vi "convert spotfield to WF.vi"(8 "error in (no error)":errorcluster, 10 "TDK-Lambda Z in":refnum<class "ThorlabsWFS.lvclass">, 11 "VISA Refnum in":refnum<visa-resource-name>) -> (0 "error out":errorcluster, 1 "output cluster":T1, 2 "Array Wavefront":sgl[](array[numeric]), 3 "VISA Refnum out":refnum<visa-resource-name>)   [LabVIEW 2020, in "ThorlabsWFS.lvclass"]
uses:
  ThorlabsWFS.lvclass
  analysis result.ctl
  OnOffTypeDef.ctl
  ThorlabsWFS.lvclass/ThorlabsWFS.ctl
panel:
  in  "analysis result":T1
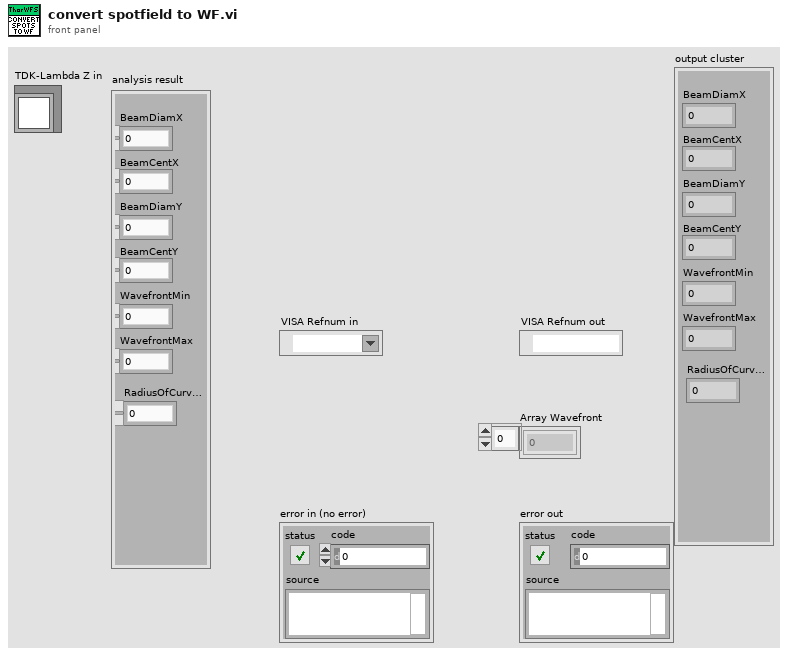
[diagram p1: front panel]
types:
  T1 = typedef "ThorlabsWFS.lvclass/analysis result.ctl" = cluster{"BeamDiamX":dbl, "BeamCentX":dbl, "BeamDiamY":dbl, "BeamCentY":dbl, "WavefrontMin":dbl, "WavefrontMax":dbl, "RadiusOfCurvature":dbl}
  T2 = typedef "OnOffTypeDef.ctl" = enum16{"off", "on"}
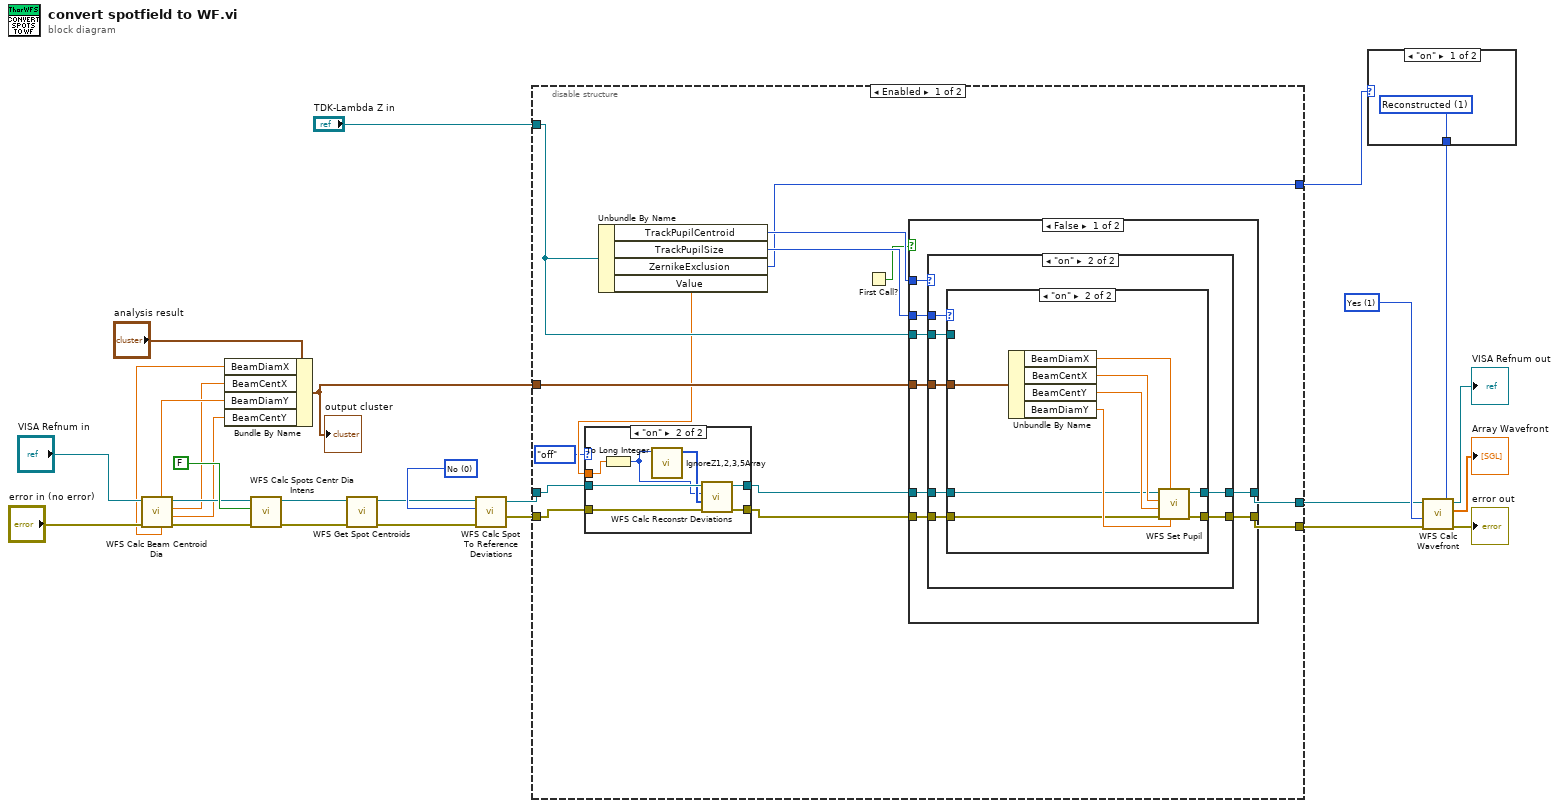
[diagram p0: block diagram]
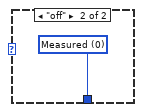
[diagram p2: hidden frame]
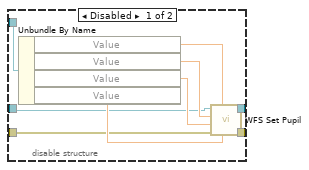
[diagram p5: hidden frame]
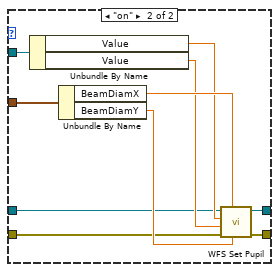
[diagram p6: hidden frame]
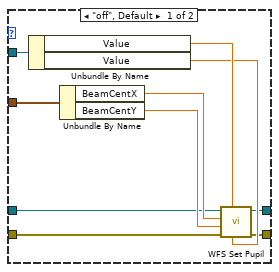
[diagram p7: hidden frame]
diagram:
  w25 = 1 items=["Yes"=1, "No"=0] ("Limit to Pupil (No)")
  w22 = 0 items=["No", "Yes"] ("Cancel Wavefront Tilt (No)")
  n1 = call "WFS Calc Beam Centroid Dia.vi"("error in (no error)"="error in (no error)", "instrument handle"="VISA Refnum in") -> ("error out"=w13:errorcluster, "Beam Centroid Y mm"=w9:dbl, "Beam Centroid X mm"=w8:dbl, "instrument handle out"=w12:refnum<visa-resource-name>, "Beam Diameter X mm"=w10:dbl, "Beam Diameter Y mm"=w11:dbl)  [unwired: 4 in]
  n2 = Bundle By Name(cluster="analysis result", "BeamDiamX"=w10, "BeamCentX"=w8, "BeamDiamY"=w11, "BeamCentY"=w9) -> (w7:T1)
  "output cluster" <- w7
  n3 = call "WFS Calc Spots Centr Dia Intens.vi"("error in (no error)"=w13, "Dynamic Noise Cut (On)"=FALSE, "instrument handle"=w12) -> ("error out"=w18:errorcluster, "instrument handle out"=w17:refnum<visa-resource-name>)  [unwired: 7 in]
  n4 = call "WFS Get Spot Centroids.vi"("error in (no error)"=w18, "instrument handle"=w17) -> ("error out"=w21:errorcluster, "instrument handle out"=w20:refnum<visa-resource-name>)  [unwired: 6 in, 2 out]
  n5 = call "WFS Calc Spot To Reference Deviations.vi"("error in (no error)"=w21, "Cancel Wavefront Tilt (No)"=w22, "instrument handle"=w20) -> ("error out"=w3:errorcluster, "instrument handle out"=w5:refnum<visa-resource-name>)  [unwired: 7 in]
  n6 = disable-structure shown="Enabled" {
    disable-tunnel: w7 -> [w38 _]
    disable-tunnel: "TDK-Lambda Z in" -> [w37 _]
    disable-tunnel: w5 -> [w34 w121]
    disable-tunnel: [w36 w121] -> w4
    disable-tunnel: w3 -> [w33 w120]
    disable-tunnel: [w35 w120] -> w2
    disable-tunnel: [w29 _] -> w1
    frame Enabled {
      n7 = Unbundle By Name(w37) -> ("TrackPupilCentroid"=w41:T2, "TrackPupilSize"=w40:T2, "ZernikeExclusion"=w29:T2, "Value"=w30:dbl)
      n8 = case shown="\"on\"" OnOffTypeDef."off" ("IgnoreZ1,2,3,5") {
        tunnel: w34 -> [w43 w50]
        tunnel: w33 -> [w42 w49]
        tunnel: [w42 w48] -> w32
        tunnel: [w43 w47] -> w31
        tunnel: w30 -> [_ w45]
        frame "off", Default {
        }
        frame "on" {
          n9 = To Long Integer(number=w45) -> (32bit integer=w44:i32)
          n10 = call "IgnoreZ1,2,3,5Array.vi"("Zernike Order"=w44) -> ("output array"=w46:i32[])  [unwired: 10 in]
          n11 = call "WFS Calc Reconstr Deviations.vi"("error in (no error)"=w49, "Array Zernike Reconstruct"=w46, "Zernike Orders"=w44, "instrument handle"=w50) -> ("error out"=w48:errorcluster, "instrument handle out"=w47:refnum<visa-resource-name>)  [unwired: 4 in, 2 out]
        }
      }
      n12 = First Call?() -> (First Call?: T/F=w39:bool)
      n13 = case shown="False" w39 {
        tunnel: w41 -> [w58 _]
        tunnel: w40 -> [w57 _]
        tunnel: w38 -> [w56 _]
        tunnel: w37 -> [w55 _]
        tunnel: w31 -> [w54 w119]
        tunnel: [w53 w119] -> w36
        tunnel: w32 -> [w52 w118]
        tunnel: [w51 w118] -> w35
        frame False {
          n14 = case shown="\"on\"" w58 {
            tunnel: w57 -> [w65 w98]
            tunnel: w56 -> [w64 w97]
            tunnel: w55 -> [w63 w96]
            tunnel: w54 -> [w62 w95]
            tunnel: [w61 w94] -> w53
            tunnel: w52 -> [w60 w93]
            tunnel: [w59 w92] -> w51
            frame "off", Default {
              n15 = case shown="\"off\", Default" w65 {
                tunnel: w64 -> [_ w91]
                tunnel: w63 -> [w70 w88]
                tunnel: w62 -> [w69 w85]
                tunnel: [w68 w84] -> w61
                tunnel: w60 -> [w67 w83]
                tunnel: [w66 w82] -> w59
                frame "off", Default {
                  n16 = disable-structure shown="Enabled" {
                    disable-tunnel: w70 -> [w79 _]
                    disable-tunnel: w69 -> [w74 w81]
                    disable-tunnel: [w73 w81] -> w68
                    disable-tunnel: w67 -> [w72 w80]
                    disable-tunnel: [w71 w80] -> w66
                    frame Disabled {
                      n17 = Unbundle By Name(w79) -> ("Value"=w78:dbl, "Value"=w76:dbl, "Value"=w75:dbl, "Value"=w77:dbl)
                      n18 = call "WFS Set Pupil.vi"("Pupil Diameter Y mm"=w77, "Pupil Diameter X mm"=w78, "error in (no error)"=w72, "Pupil Center Y mm"=w75, "Pupil Center X mm"=w76, "instrument handle"=w74) -> ("error out"=w71:errorcluster, "instrument handle out"=w73:refnum<visa-resource-name>)  [unwired: 4 in]
                    }
                    frame Enabled {
                    }
                  }
                }
                frame "on" {
                  n19 = Unbundle By Name(w88) -> ("Value"=w87:dbl, "Value"=w86:dbl)
                  n20 = Unbundle By Name(w91) -> ("BeamDiamX"=w90:dbl, "BeamDiamY"=w89:dbl)
                  n21 = call "WFS Set Pupil.vi"("Pupil Diameter Y mm"=w89, "Pupil Diameter X mm"=w90, "error in (no error)"=w83, "Pupil Center Y mm"=w86, "Pupil Center X mm"=w87, "instrument handle"=w85) -> ("error out"=w82:errorcluster, "instrument handle out"=w84:refnum<visa-resource-name>)  [unwired: 4 in]
                }
              }
            }
            frame "on" {
              n22 = case shown="\"on\"" w98 {
                tunnel: w97 -> [w106 w117]
                tunnel: w96 -> [w105 _]
                tunnel: w95 -> [w102 w109]
                tunnel: [w101 w112] -> w94
                tunnel: w93 -> [w100 w110]
                tunnel: [w99 w111] -> w92
                frame "off", Default {
                  n23 = Unbundle By Name(w105) -> ("Value"=w104:dbl, "Value"=w103:dbl)
                  n24 = Unbundle By Name(w106) -> ("BeamCentX"=w108:dbl, "BeamCentY"=w107:dbl)
                  n25 = call "WFS Set Pupil.vi"("Pupil Diameter Y mm"=w103, "Pupil Diameter X mm"=w104, "error in (no error)"=w100, "Pupil Center Y mm"=w107, "Pupil Center X mm"=w108, "instrument handle"=w102) -> ("error out"=w99:errorcluster, "instrument handle out"=w101:refnum<visa-resource-name>)  [unwired: 4 in]
                }
                frame "on" {
                  n26 = Unbundle By Name(w117) -> ("BeamDiamX"=w116:dbl, "BeamCentX"=w115:dbl, "BeamCentY"=w113:dbl, "BeamDiamY"=w114:dbl)
                  n27 = call "WFS Set Pupil.vi"("Pupil Diameter Y mm"=w114, "Pupil Diameter X mm"=w116, "error in (no error)"=w110, "Pupil Center Y mm"=w113, "Pupil Center X mm"=w115, "instrument handle"=w109) -> ("error out"=w111:errorcluster, "instrument handle out"=w112:refnum<visa-resource-name>)  [unwired: 4 in]
                }
              }
            }
          }
        }
        frame True {
        }
      }
    }
    frame Disabled {
    }
  }
  n28 = case shown="\"on\"" w1 {
    tunnel: [w122 w123] -> w26
    frame "on" {
      w122 = 1 items=["Measured", "Reconstructed", "Difference"] ("Wavefront Type (Measured)")
    }
    frame "off" {
      w123 = 0 items=["Measured", "Reconstructed", "Difference"] ("Wavefront Type (Measured)")
    }
  }
  n29 = call "WFS Calc Wavefront.vi"("error in (no error)"=w2, "Limit to Pupil (No)"=w25, "Wavefront Type (Measured)"=w26, "instrument handle"=w4) -> ("error out"=→"error out":errorcluster, "Array Wavefront"=→"Array Wavefront":sgl[], "instrument handle out"=→"VISA Refnum out":refnum<visa-resource-name>)  [unwired: 5 in]
